vi "ListenForEcho.vi"(8 "error in (no error)":errorcluster, 9 "Tx Array":u8[](array[numeric]), 11 "milliseconds to wait":u32) -> (0 "error out":errorcluster, 2 "Success?":bool)   [LabVIEW 2013]
uses:
  RxTx/XceiverStates.ctl
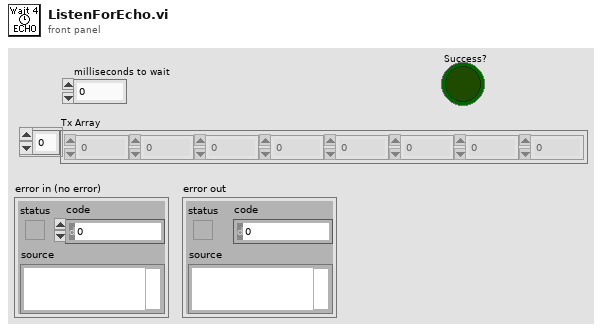
[diagram p1: front panel]
types:
  T1 = typedef "XceiverStates.ctl" = enum16{"Initialize", "Rx", "Tx", "Raw Mode", "Clear Buffer", "ClearEcho", "Read Buffer", "Close"}
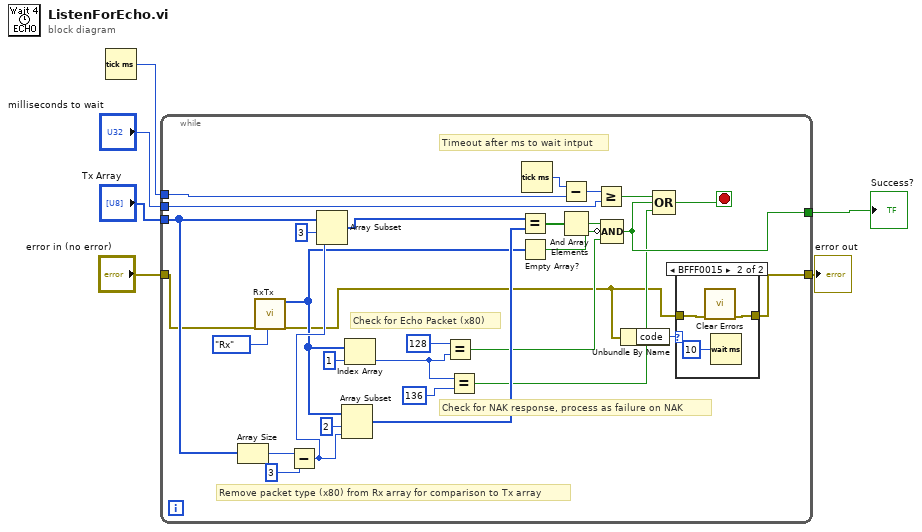
[diagram p0: block diagram]
diagram:
  n1 = Tick Count (ms)() -> (millisecond timer value=w5:u32)
  n2 = while {
    tunnel: "Tx Array" -> [w23]
    tunnel: w5 -> [w35]
    tunnel: "error in (no error)" -> [w20]
    tunnel: [w9] -> w3
    tunnel: "milliseconds to wait" -> [w30]
    tunnel: [w12] -> w1
    stop <- w10 stop-if-true
    # "Check for NAK response, process as failure on NAK"
    # "Remove packet type (x80) from Rx array for comparison to Tx array"
    # "Check for Echo Packet (x80)"
    # "Timeout after ms to wait intput"
    n3 = Array Size(array=w23) -> (size(s)=w26:i32)
    n4 = call "RxTx.vi"("error in (no error)"=w20, "Action"=XceiverStates."Rx") -> ("[Raw RxData]"=w17:u8[], "error out"=w8:errorcluster)  [unwired: 9 in, 7 out]
    n5 = Subtract(x=w26, y=3) -> (x-y=w19:i32)
    n6 = Array Subset(array=w23, index=3, length=w19) -> (w22:u8[])
    n7 = Array Subset(array=w17, index=2, length=w19) -> (w24:u8[])
    n8 = Index Array(array=w17, index=1) -> (element=w15:u8)
    n9 = Equal?(x=u8 128, y=w15) -> (x = y?=w18:bool)
    n10 = Equal?(x=w15, y=u8 136) -> (x = y?=w11:bool)
    n11 = Equal?(x=w22, y=w24) -> (x = y?=w33:bool[])
    n12 = Empty Array?(array=w17) -> (empty?=w31:bool)
    n13 = Tick Count (ms)() -> (millisecond timer value=w36:u32)
    n14 = Subtract(x=w36, y=w35) -> (x-y=w29:u32)
    n15 = And Array Elements(Boolean array=w33) -> (logical AND=w32:bool)
    n16 = Greater Or Equal?(x=w29, y=w30) -> (x >= y?=w13:bool)
    n17 = Compound Arithmetic op=AND(w32, invert w31, w18) -> (w12:bool)
    n18 = Unbundle By Name(w8) -> ("code"=w7:i32)
    n19 = Compound Arithmetic op=OR(w13, w12, w11) -> (w10:bool)
    n20 = case shown="BFFF0015" w7 {
      tunnel: [w37 w40] -> w9
      tunnel: w8 -> [w37 w38]
      frame Default {
      }
      frame -1073807339 {
        n21 = call <vilib>:"Clear Errors.vi"("error in (no error)"=w38) -> ("error out"=w40:errorcluster)  [unwired: 6 in]
        n22 = Wait (ms)(milliseconds to wait=u32 10) -> ()  [unwired: 1 out]
      }
    }
  }
  "error out" <- w3
  "Success?" <- w1
